vi "Hahn & RF no pi Pulse Sequence Generator.vi"(0 "N Loop":i32=10000, 1 "Rabi Frequency":dbl, 2 "RF Pulse":dbl, 3 "Tau":dbl, 5 "AOM Pulse length":dbl=2.5e-06, 7 "AOM Rest time":dbl=1e-06, 9 "Signal Delay":dbl=6e-07, 11 "APD signal width":dbl=5e-07, 12 "MW Delay":dbl, 13 "Pulse offset":dbl) -> (4 "Pulse Sequence":T1(array[cluster]))   [LabVIEW 2012]
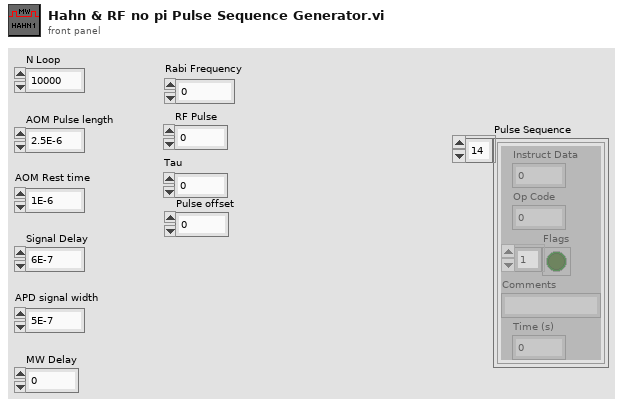
[diagram p1: front panel]
types:
  T1 = cluster{"Instruct Data":i32, "Op Code":i32, "Flags":bool[], "Comments":string, "Time (s)":dbl}[]
  T2 = cluster{"Instruct Data":i32, "Op Code":i32, "Flags":bool[], "Comments":string, "Time (s)":dbl}
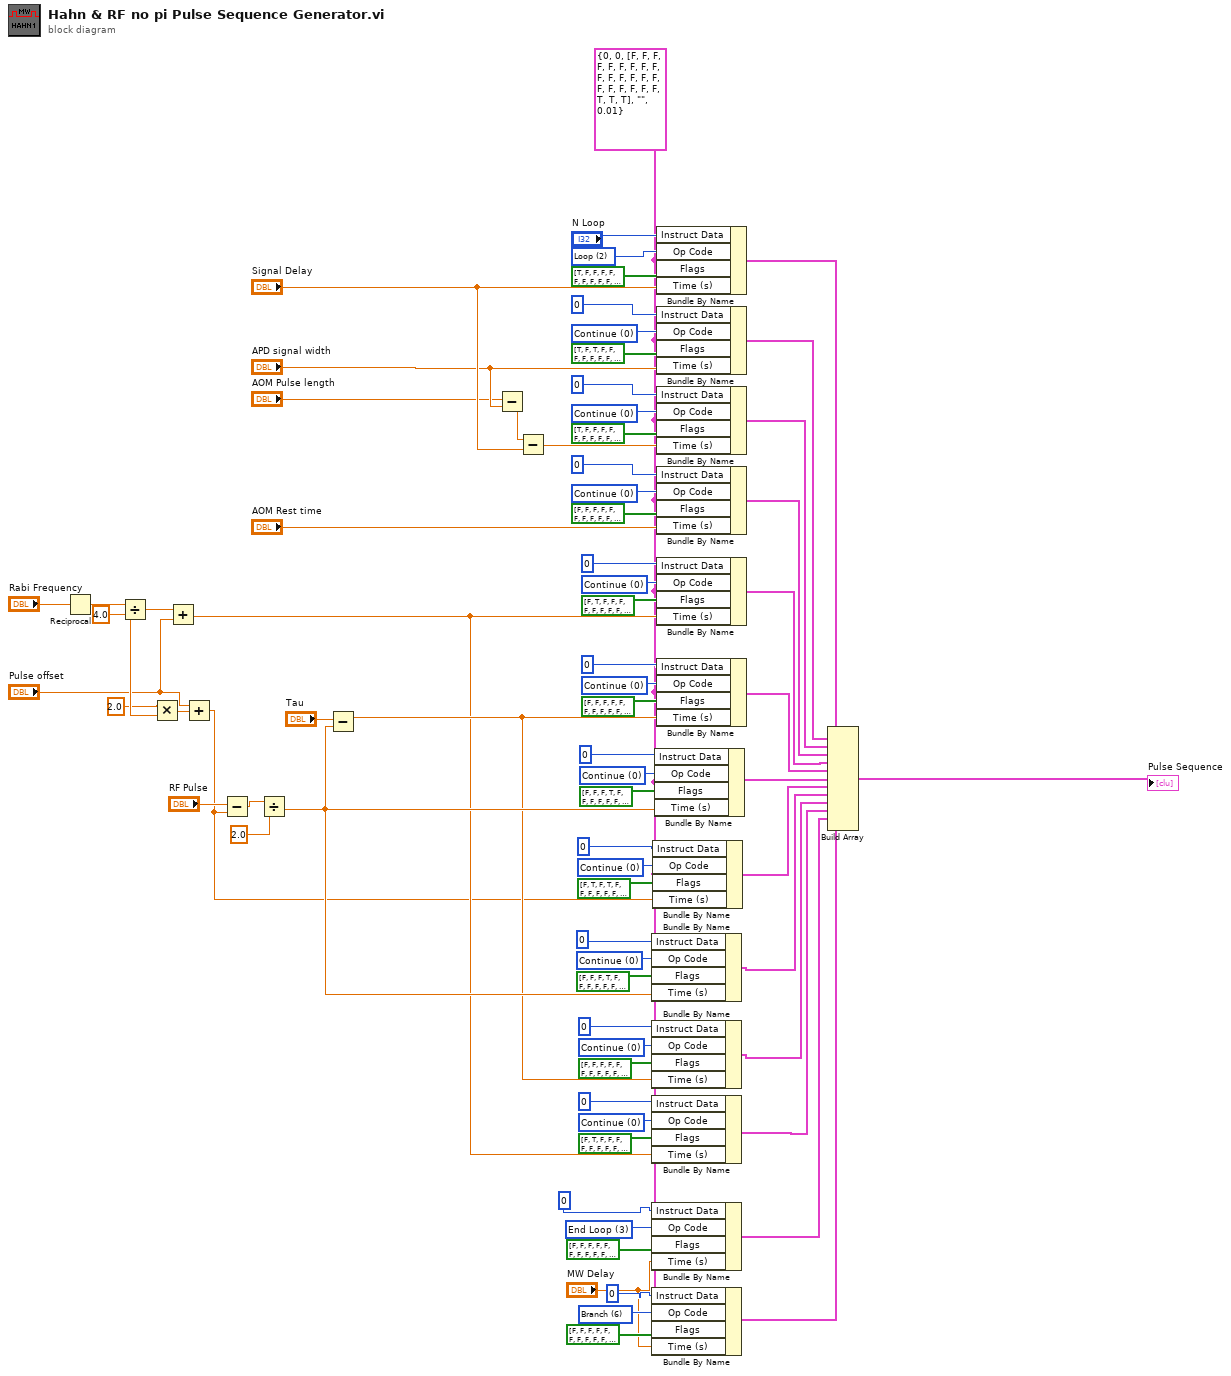
[diagram p0: block diagram]
diagram:
  w6 = 6 items=["Continue", "Stop", "Loop", "End Loop", "JSR", "RTS", "Branch", "Long Delay", "Wait"] ("Op Code")
  w21 = 0 items=["Continue", "Stop", "Loop", "End Loop", "JSR", "RTS", "Branch", "Long Delay", "Wait"] ("Op Code")
  w24 = 0 items=["Continue", "Stop", "Loop", "End Loop", "JSR", "RTS", "Branch", "Long Delay", "Wait"] ("Op Code")
  w33 = 0 items=["Continue", "Stop", "Loop", "End Loop", "JSR", "RTS", "Branch", "Long Delay", "Wait"] ("Op Code")
  w36 = 0 items=["Continue", "Stop", "Loop", "End Loop", "JSR", "RTS", "Branch", "Long Delay", "Wait"] ("Op Code")
  w40 = 0 items=["Continue", "Stop", "Loop", "End Loop", "JSR", "RTS", "Branch", "Long Delay", "Wait"] ("Op Code")
  w43 = 0 items=["Continue", "Stop", "Loop", "End Loop", "JSR", "RTS", "Branch", "Long Delay", "Wait"] ("Op Code")
  w46 = 0 items=["Continue", "Stop", "Loop", "End Loop", "JSR", "RTS", "Branch", "Long Delay", "Wait"] ("Op Code")
  w57 = 3 items=["Continue", "Stop", "Loop", "End Loop", "JSR", "RTS", "Branch", "Long Delay", "Wait"] ("Op Code")
  w62 = 0 items=["Continue", "Stop", "Loop", "End Loop", "JSR", "RTS", "Branch", "Long Delay", "Wait"] ("Op Code")
  w66 = 0 items=["Continue", "Stop", "Loop", "End Loop", "JSR", "RTS", "Branch", "Long Delay", "Wait"] ("Op Code")
  w69 = 0 items=["Continue", "Stop", "Loop", "End Loop", "JSR", "RTS", "Branch", "Long Delay", "Wait"] ("Op Code")
  w71 = 2 items=["Continue", "Stop", "Loop", "End Loop", "JSR", "RTS", "Branch", "Long Delay", "Wait"] ("Op Code")
  w3 = T2 {"Instruct Data"=0, "Op Code"=0, "Flags"=[FALSE, FALSE, FALSE, FALSE, FALSE, FALSE, FALSE, FALSE, FALSE, FALSE, FALSE, FALSE, FALSE, FALSE, FALSE, FALSE, FALSE, FALSE, FALSE, FALSE, FALSE, TRUE, TRUE, TRUE], "Comments"="", "Time (s)"=0.01} ("PB Inst 2")
  n1 = Reciprocal(x="Rabi Frequency") -> (1/x=w51:dbl)
  n2 = Divide(x=w51, y=4.0) -> (x/y=w50:dbl)
  n3 = Multiply(x=2.0, y=w50) -> (x*y=w38:dbl)
  n4 = Add(x=w50, y="Pulse offset") -> (x+y=w10:dbl)
  n5 = Add(x="Pulse offset", y=w38) -> (x+y=w9:dbl)
  n6 = Subtract(x="RF Pulse", y=w9) -> (x-y=w29:dbl)
  n7 = Divide(x=w29, y=2.0) -> (x/y=w26:dbl)
  n8 = Subtract(x="Tau", y=w26) -> (x-y=w19:dbl)
  n9 = Subtract(x="AOM Pulse length", y="APD signal width") -> (x-y=w64:dbl)
  n10 = Subtract(x=w64, y="Signal Delay") -> (x-y=w60:dbl)
  n11 = Bundle By Name(cluster=w3, "Instruct Data"=0, "Op Code"=w33, "Flags"=bool[] [FALSE, FALSE, FALSE, TRUE, FALSE, FALSE, FALSE, FALSE, FALSE, FALSE, FALSE, FALSE, FALSE, FALSE, FALSE, FALSE, FALSE, FALSE, FALSE, FALSE, FALSE, TRUE, TRUE, TRUE], "Time (s)"=w26) -> (w13:T2)
  n12 = Bundle By Name(cluster=w3, "Instruct Data"=0, "Op Code"=w24, "Flags"=bool[] [FALSE, FALSE, FALSE, FALSE, FALSE, FALSE, FALSE, FALSE, FALSE, FALSE, FALSE, FALSE, FALSE, FALSE, FALSE, FALSE, FALSE, FALSE, FALSE, FALSE, FALSE, TRUE, TRUE, TRUE], "Time (s)"=w19) -> (w12:T2)
  n13 = Bundle By Name(cluster=w3, "Instruct Data"=0, "Op Code"=w21, "Flags"=bool[] [FALSE, TRUE, FALSE, FALSE, FALSE, FALSE, FALSE, FALSE, FALSE, FALSE, FALSE, FALSE, FALSE, FALSE, FALSE, FALSE, FALSE, FALSE, FALSE, FALSE, FALSE, TRUE, TRUE, TRUE], "Time (s)"=w10) -> (w11:T2)
  n14 = Bundle By Name(cluster=w3, "Instruct Data"=0 ("y"), "Op Code"=w57, "Flags"=bool[] [FALSE, FALSE, FALSE, FALSE, FALSE, FALSE, FALSE, FALSE, FALSE, FALSE, FALSE, FALSE, FALSE, FALSE, FALSE, FALSE, FALSE, FALSE, FALSE, FALSE, FALSE, TRUE, TRUE, TRUE], "Time (s)"="MW Delay") -> (w8:T2)
  n15 = Bundle By Name(cluster=w3, "Instruct Data"=0 ("y"), "Op Code"=w6, "Flags"=bool[] [FALSE, FALSE, FALSE, FALSE, FALSE, FALSE, FALSE, FALSE, FALSE, FALSE, FALSE, FALSE, FALSE, FALSE, FALSE, FALSE, FALSE, FALSE, FALSE, FALSE, FALSE, TRUE, TRUE, TRUE], "Time (s)"="MW Delay") -> (w2:T2)
  n16 = Bundle By Name(cluster=w3, "Instruct Data"=0, "Op Code"=w36, "Flags"=bool[] [FALSE, TRUE, FALSE, TRUE, FALSE, FALSE, FALSE, FALSE, FALSE, FALSE, FALSE, FALSE, FALSE, FALSE, FALSE, FALSE, FALSE, FALSE, FALSE, FALSE, FALSE, TRUE, TRUE, TRUE], "Time (s)"=w9) -> (w14:T2)
  n17 = Bundle By Name(cluster=w3, "Instruct Data"=0, "Op Code"=w40, "Flags"=bool[] [FALSE, FALSE, FALSE, TRUE, FALSE, FALSE, FALSE, FALSE, FALSE, FALSE, FALSE, FALSE, FALSE, FALSE, FALSE, FALSE, FALSE, FALSE, FALSE, FALSE, FALSE, TRUE, TRUE, TRUE], "Time (s)"=w26) -> (w15:T2)
  n18 = Bundle By Name(cluster=w3, "Instruct Data"="N Loop", "Op Code"=w71, "Flags"=bool[] [TRUE, FALSE, FALSE, FALSE, FALSE, FALSE, FALSE, FALSE, FALSE, FALSE, FALSE, FALSE, FALSE, FALSE, FALSE, FALSE, FALSE, FALSE, FALSE, FALSE, FALSE, TRUE, TRUE, TRUE], "Time (s)"="Signal Delay") -> (w56:T2)
  n19 = Bundle By Name(cluster=w3, "Instruct Data"=0, "Op Code"=w69, "Flags"=bool[] [TRUE, FALSE, TRUE, FALSE, FALSE, FALSE, FALSE, FALSE, FALSE, FALSE, FALSE, FALSE, FALSE, FALSE, FALSE, FALSE, FALSE, FALSE, FALSE, FALSE, FALSE, TRUE, TRUE, TRUE], "Time (s)"="APD signal width") -> (w55:T2)
  n20 = Bundle By Name(cluster=w3, "Instruct Data"=0, "Op Code"=w66, "Flags"=bool[] [TRUE, FALSE, FALSE, FALSE, FALSE, FALSE, FALSE, FALSE, FALSE, FALSE, FALSE, FALSE, FALSE, FALSE, FALSE, FALSE, FALSE, FALSE, FALSE, FALSE, FALSE, TRUE, TRUE, TRUE], "Time (s)"=w60) -> (w54:T2)
  n21 = Bundle By Name(cluster=w3, "Instruct Data"=0, "Op Code"=w62, "Flags"=bool[] [FALSE, FALSE, FALSE, FALSE, FALSE, FALSE, FALSE, FALSE, FALSE, FALSE, FALSE, FALSE, FALSE, FALSE, FALSE, FALSE, FALSE, FALSE, FALSE, FALSE, FALSE, TRUE, TRUE, TRUE], "Time (s)"="AOM Rest time") -> (w53:T2)
  n22 = Bundle By Name(cluster=w3, "Instruct Data"=0, "Op Code"=w46, "Flags"=bool[] [FALSE, TRUE, FALSE, FALSE, FALSE, FALSE, FALSE, FALSE, FALSE, FALSE, FALSE, FALSE, FALSE, FALSE, FALSE, FALSE, FALSE, FALSE, FALSE, FALSE, FALSE, TRUE, TRUE, TRUE], "Time (s)"=w10) -> (w17:T2)
  n23 = Bundle By Name(cluster=w3, "Instruct Data"=0, "Op Code"=w43, "Flags"=bool[] [FALSE, FALSE, FALSE, FALSE, FALSE, FALSE, FALSE, FALSE, FALSE, FALSE, FALSE, FALSE, FALSE, FALSE, FALSE, FALSE, FALSE, FALSE, FALSE, FALSE, FALSE, TRUE, TRUE, TRUE], "Time (s)"=w19) -> (w16:T2)
  n24 = Build Array(w56, w55, w54, w53, w17, w16, w15, w14, w13, w12, w11, w8, w2) -> (→"Pulse Sequence":T1)
